vi "Initialize Actor.vi"(7 "Host Name":string, 8 "error in (no error)":errorcluster, 9 "Actor Name":string, 10 "Message Broker Interface":refnum<class "Message Broker Interface.lvclass">, 11 "Mediated Actor in":refnum<class "Mediated Actor.lvclass">) -> (0 "error out":errorcluster, 3 "Mediated Actor out":refnum<class "Mediated Actor.lvclass">)   [LabVIEW 2016, in "Stream Mediator.lvlib" / "Mediated Actor.lvclass"]
doc: "--\nCopyright © 2017 Composed SystemsI All rights reserved.\n\nAuthor: Jon McBee <jon.mcbee@composed.io>\n\nThis library is provided \"AS IS\" ,WITHOUT WARRANTIES OR\nCONDITIONS OF ANY KIND, either express or implied.\n\nComposed Systems -- composed.io\n\nStream 0.0.1.1\nJon McBee - Composed Systems\nCopyright (c) 2017, Composed Systems"
uses:
  <userlib>/Composed Systems/Stream/Mediator/Classes/Mediated Actor/Mediated Actor.lvclass
  <userlib>/Composed Systems/Stream/Mediator/Classes/Message Broker Interface/Message Broker Interface.lvclass
  <userlib>/Composed Systems/Stream/Mediator/Classes/Message Transport Queue/Message Transport Queue.lvclass
  <userlib>/Composed Systems/Stream/Mediator/Classes/Mediated Actor/Mediated Actor.lvclass/Mediated Actor.ctl
  <userlib>/Composed Systems/Stream/Mediator/Classes/Message Transport Event/Message Transport Event.lvclass
  C:/Program Files (x86)/National Instruments/LabVIEW 2016/user.lib/Composed Systems/Stream/Mediator/Classes/Message Transport Interface/Message Transport Interface.lvclass
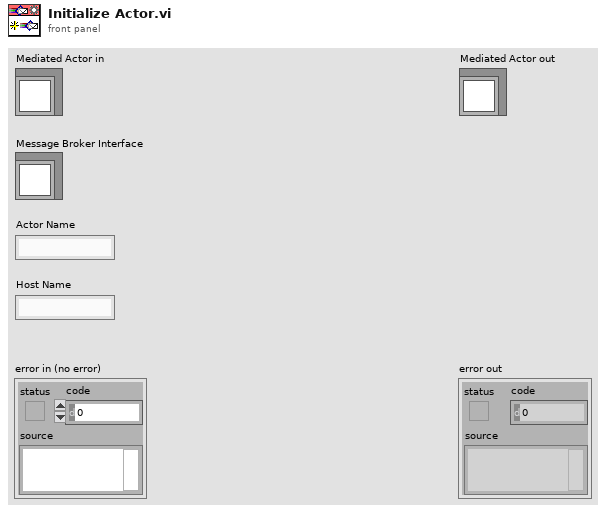
[diagram p1: front panel]
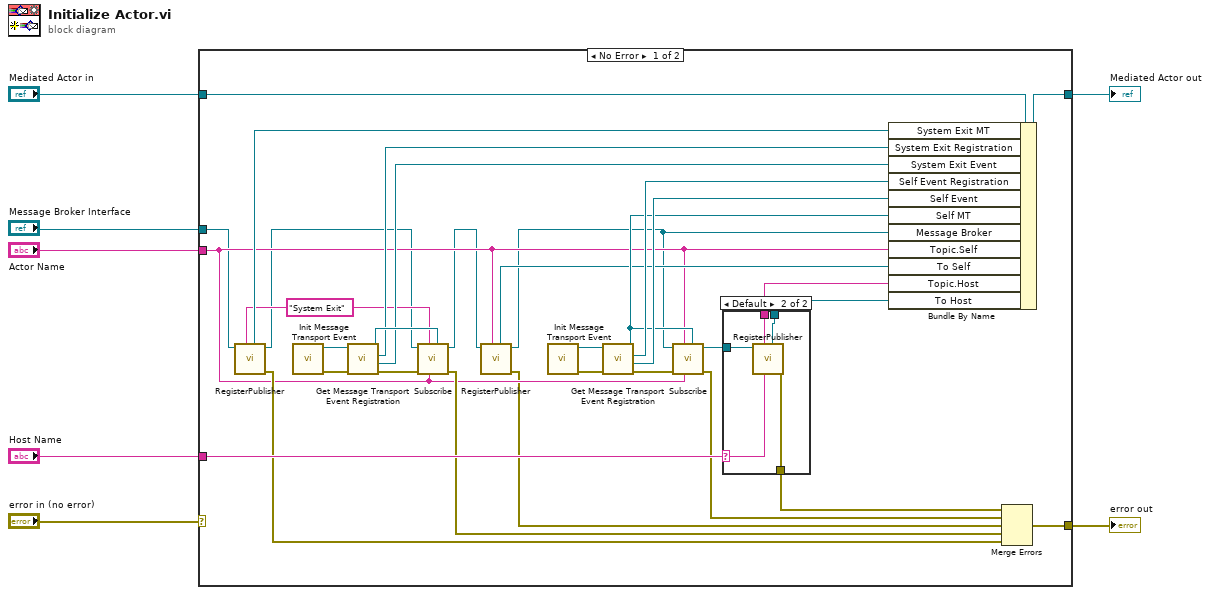
[diagram p0: block diagram]
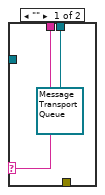
[diagram p2: hidden frame]
diagram:
  n1 = case shown="No Error" "error in (no error)" {
    selector: "error in (no error)" -> [_ w47]
    tunnel: [w27 w47] -> w6
    tunnel: [w39 w46] -> w4
    tunnel: "Mediated Actor in" -> [w26 w46]
    tunnel: "Message Broker Interface" -> [w14 _]
    tunnel: "Actor Name" -> [w15 _]
    tunnel: "Host Name" -> [w28 _]
    frame No Error {
      w17 = "System Exit" ("Topic Name")
      n2 = call-dynamic "RegisterPublisher.vi"("Topic Name"=w17, "Message Broker Interface in"=w14) -> ("error out"=w16:errorcluster, "Message Broker Interface out"=w13:refnum<class "Message Broker Interface.lvclass">, "Transport"=w18:refnum<class "Message Transport Queue.lvclass">)  [unwired: 5 in, 2 out]
      n3 = call <userlib>:"Init Message Transport Event.vi"() -> ("error out"=w22:errorcluster, "Message Transport Event out"=w23:refnum<class "Message Transport Event.lvclass">)  [unwired: 10 in]
      n4 = call <userlib>:"Get Message Transport Event Registration.vi"("error in (no error)"=w22, "Message Transport Event in"=w23) -> ("error out"=w24:errorcluster, "Event"=w19:refnum<user-event>, "Event Registration Refnum"=w20:refnum<event-registration>, "Message Transport Event out"=w25:refnum<class "Message Transport Event.lvclass">)  [unwired: 6 in]
      n5 = call-dynamic "Subscribe.vi"("Message Transport Interface"=w25, "Subscriber Name"=w15, "Topic Name"=w17, "error in (no error)"=w24, "Message Broker Interface in"=w13) -> ("error out"=w21:errorcluster, "Message Broker Interface out"=w11:refnum<class "Message Broker Interface.lvclass">)  [unwired: 4 in, 1 out]
      n6 = call-dynamic "RegisterPublisher.vi"("Topic Name"=w15, "Message Broker Interface in"=w11) -> ("error out"=w9:errorcluster, "Message Broker Interface out"=w10:refnum<class "Message Broker Interface.lvclass">, "Transport"=w31:refnum<class "Message Transport Queue.lvclass">)  [unwired: 5 in, 2 out]
      n7 = call <userlib>:"Init Message Transport Event.vi"() -> ("error out"=w38:errorcluster, "Message Transport Event out"=w37:refnum<class "Message Transport Event.lvclass">)  [unwired: 10 in]
      n8 = call <userlib>:"Get Message Transport Event Registration.vi"("error in (no error)"=w38, "Message Transport Event in"=w37) -> ("error out"=w36:errorcluster, "Event"=w33:refnum<user-event>, "Event Registration Refnum"=w34:refnum<event-registration>, "Message Transport Event out"=w32:refnum<class "Message Transport Event.lvclass">)  [unwired: 6 in]
      n9 = call-dynamic "Subscribe.vi"("Message Transport Interface"=w32, "Subscriber Name"=w15, "Topic Name"=w15, "error in (no error)"=w36, "Message Broker Interface in"=w10) -> ("error out"=w8:errorcluster, "Message Broker Interface out"=w12:refnum<class "Message Broker Interface.lvclass">)  [unwired: 4 in, 1 out]
      n10 = case shown="Default" w28 {
        selector: w28 -> [w41 w44]
        tunnel: w12 -> [_ w45]
        tunnel: [w41 w44] -> w30
        tunnel: [refnum<class "Message Transport Queue.lvclass"> refnum ("Transport") w43] -> w29
        tunnel: [_ w42] -> w35
        frame "" {
        }
        frame Default {
          n11 = call-dynamic "RegisterPublisher.vi"("Topic Name"=w44, "Message Broker Interface in"=w45) -> ("error out"=w42:errorcluster, "Transport"=w43:refnum<class "Message Transport Queue.lvclass">)  [unwired: 5 in, 3 out]
        }
      }
      n12 = Bundle By Name(cluster=w26, "System Exit MT"=w18, "System Exit Registration"=w20, "System Exit Event"=w19, "Self Event Registration"=w34, "Self Event"=w33, "Self MT"=w32, "Message Broker"=w10, "Topic.Self"=w15, "To Self"=w31, "Topic.Host"=w30, "To Host"=w29) -> (w39:refnum<class "Mediated Actor.lvclass">)
      n13 = Merge Errors(w35, w8, w9, w21, w16) -> (w27:errorcluster)
    }
    frame Error {
    }
  }
  "error out" <- w6
  "Mediated Actor out" <- w4
